vi "Projekt3.vi"() -> ()   [LabVIEW 2026]
uses:
  <vilib>/Utility/file.llb/Read Delimited Spreadsheet (string).vi
  <vilib>/Analysis/NI_AALBase.lvlib
panel:
  out "Approach3":dbl[](array[numeric])
  out "Approach2 Min":dbl[](array[numeric])
  out "Approach1 Max":dbl[](array[numeric])
  out "array w/ subset deleted":path[](array[path])
  out "All Files in Dir":path[](array[path])
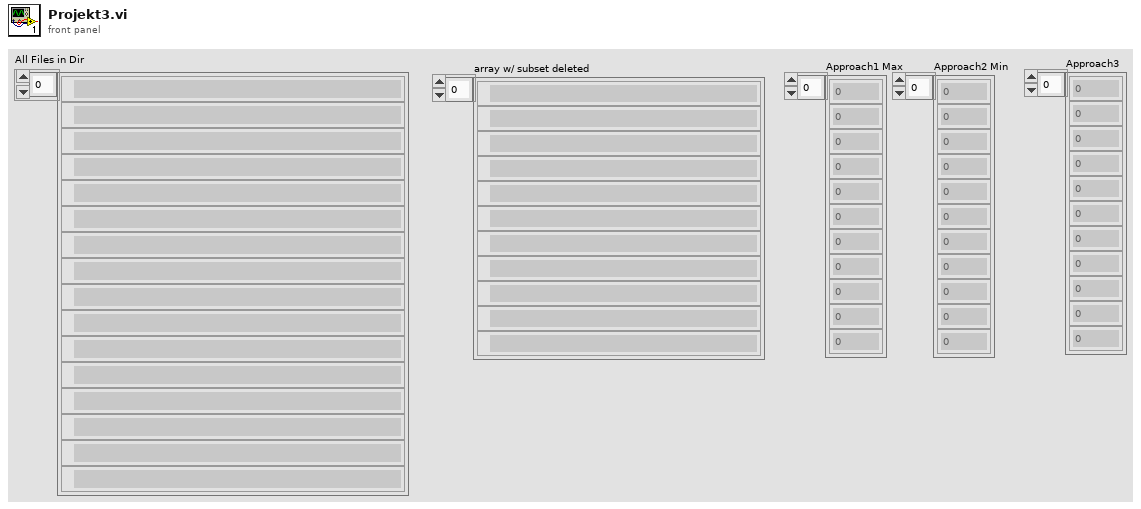
[diagram p1: front panel]
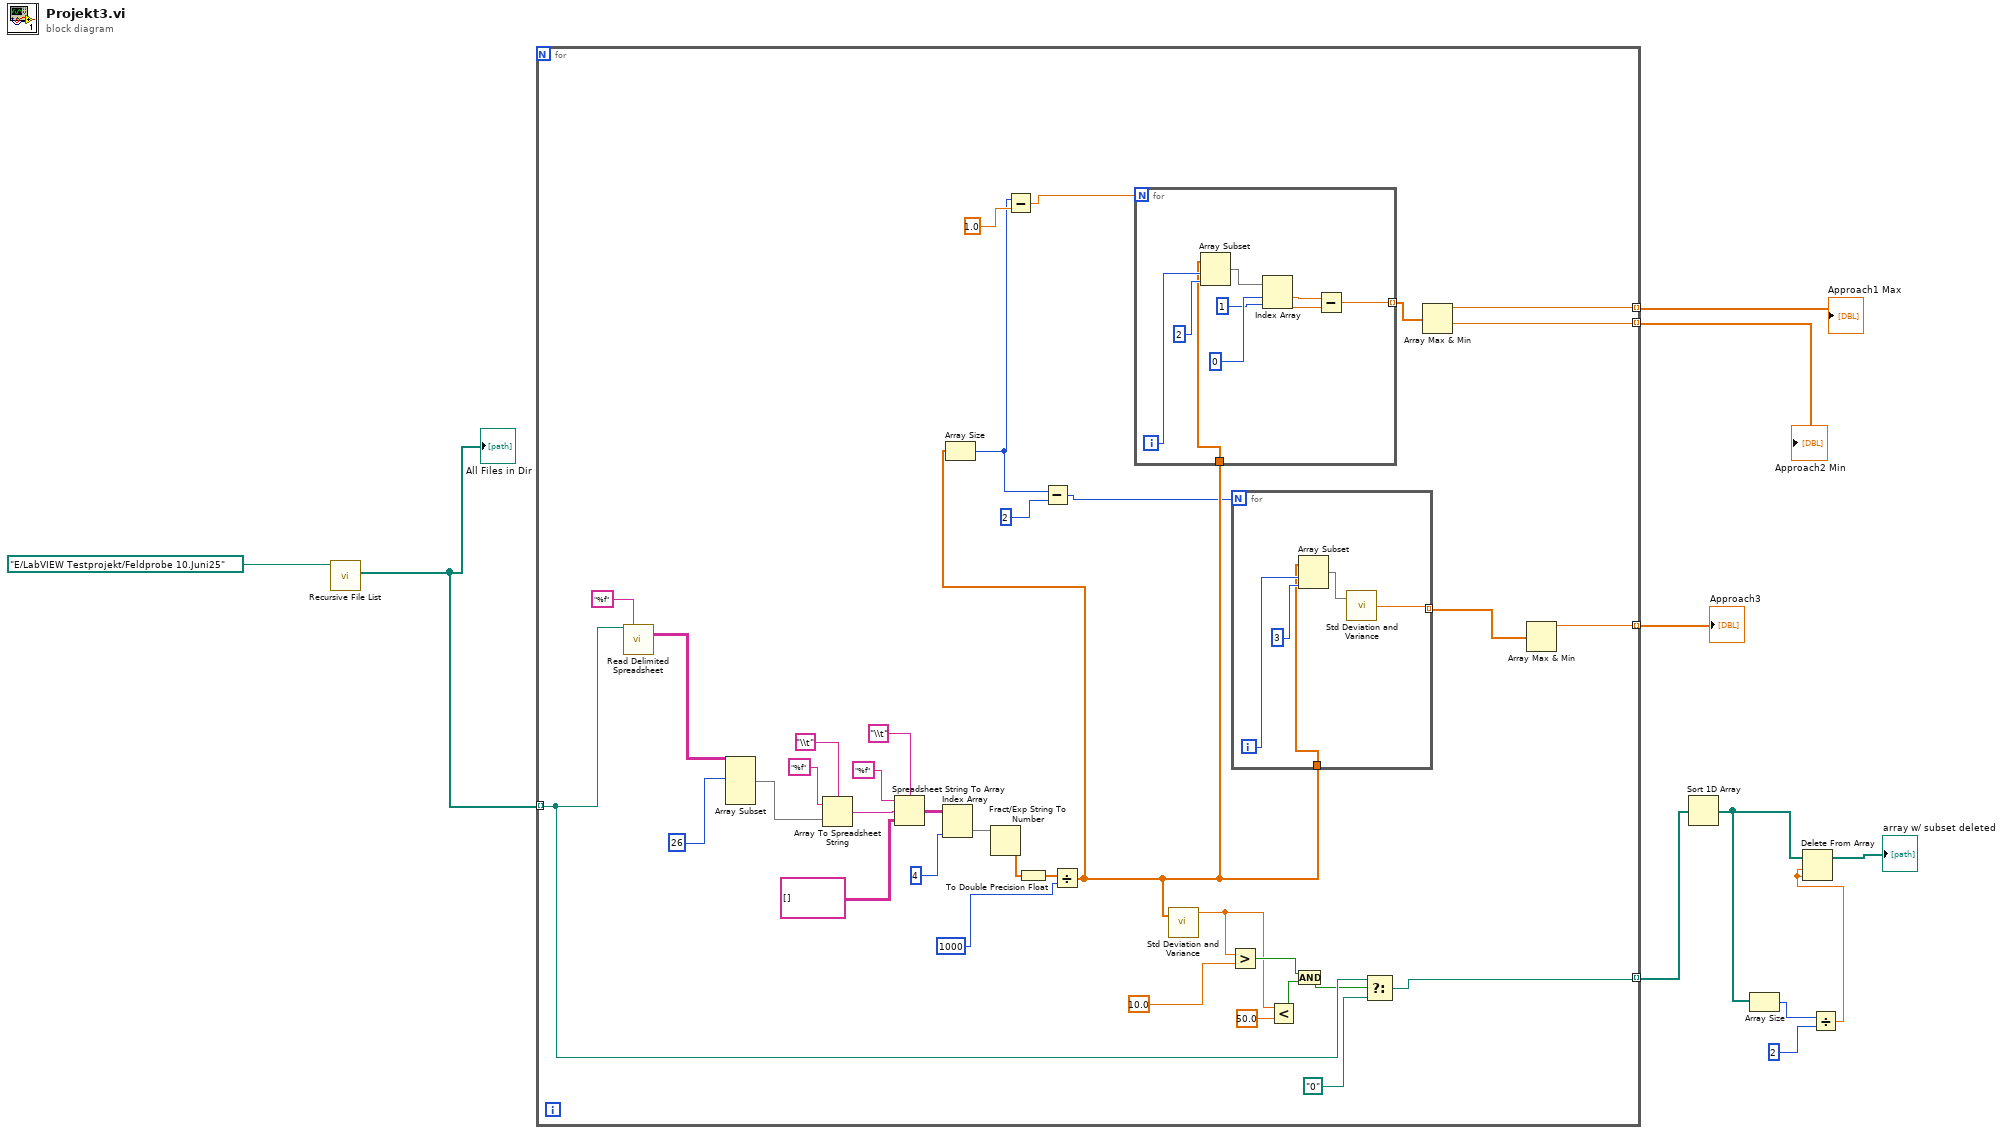
[diagram p0: block diagram]
diagram:
  n1 = call <vilib>:"Recursive File List.vi"("Folder Path"=path "E:/LabVIEW Testprojekt/Feldprobe 10.Juni25") -> ("All Files in Dir"=w10:path[])  [unwired: 6 in, 4 out]
  "All Files in Dir" <- w10
  n2 = for {
    tunnel: w10 -> [w31] mode=indexing
    tunnel: [w23] -> w9 mode=indexing
    tunnel: [w19] -> w3 mode=indexing
    tunnel: [w18] -> w2 mode=indexing
    tunnel: [w12] -> w1 mode=indexing
    n3 = call-poly <vilib>:"Read Delimited Spreadsheet.vi"("file path (dialog if empty)"=w31, "format (%s)"="%f") -> ("all rows"=w32:string[][])  [unwired: 8 in, 5 out]
    n4 = Array Subset(array=w32, index (row)=26 ("index")) -> (w44:string[][])  [unwired: 3 in]
    n5 = Array To Spreadsheet String(delimiter (Tab)="\\t", array=w44, 3:"%f" ("format string")) -> (spreadsheet string=w43:string)
    n6 = Spreadsheet String To Array(delimiter (Tab)="\\t", format string="%f", spreadsheet string=w43, array type (2D Dbl)=string[][] []) -> (array=w41:string[][])
    n7 = Index Array(array=w41, index (col)=4 ("disabled index (col)")) -> (element=w42:string[])  [unwired: 1 in]
    n8 = Fract/Exp String To Number(string=w42) -> (number=w46:dbl[])  [unwired: 3 in, 1 out]
    n9 = To Double Precision Float(number=w46) -> (double precision float=w45:dbl[])
    n10 = Divide(x=w45, y=1000) -> (x/y=w17:dbl[])
    n11 = Array Size(array=w17) -> (size(s)=w16:i32)
    n12 = Subtract(x=w16, y=1.0) -> (x-y=w21:dbl)
    n13 = Subtract(x=w16, y=2) -> (x-y=w14:i32)
    n14 = for {
      N: w21 -> [_]
      tunnel: w17 -> [w53]
      tunnel: [w55] -> w20 mode=indexing
      i -> [w54]
      n15 = Array Subset(array=w53, index=w54, length=2) -> (w60:dbl[])
      n16 = Index Array(array=w60, index #1=0 ("index"), index #2=1 ("index")) -> (element #1=w57:dbl, element #2=w56:dbl)
      n17 = Subtract(x=w57, y=w56) -> (x-y=w55:dbl)
    }
    n18 = call <vilib>:"Std Deviation and Variance.vi"("X"=w17) -> ("mean"=w27:dbl)  [unwired: 1 in, 2 out]
    n19 = Greater?(x=w27, y=10.0) -> (0:w29:bool)
    n20 = for {
      N: w14 -> [_]
      tunnel: w17 -> [w50]
      tunnel: [w48] -> w13 mode=indexing
      i -> [w51]
      n21 = Array Subset(array=w50, index=w51, length=3) -> (w49:dbl[])
      n22 = call <vilib>:"Std Deviation and Variance.vi"("X"=w49) -> ("standard deviation"=w48:dbl)  [unwired: 1 in, 2 out]
    }
    n23 = Less?(x=w27, y=50.0) -> (x < y?=w28:bool)
    n24 = And(x=w29, y=w28) -> (x .and. y?=w25:bool)
    n25 = Select(t=w31, s=w25, f=path "0") -> (s? t:f=w23:path)
    n26 = Array Max & Min(array=w20) -> (max value=w19:dbl, min value=w18:dbl)  [unwired: 2 out]
    n27 = Array Max & Min(array=w13) -> (max value=w12:dbl)  [unwired: 3 out]
  }
  "Approach1 Max" <- w3
  "Approach2 Min" <- w2
  "Approach3" <- w1
  n28 = Sort 1D Array(array=w9) -> (sorted array=w8:path[])
  n29 = Array Size(array=w8) -> (size(s)=w7:i32)
  n30 = Divide(x=w7, y=2) -> (x/y=w5:dbl)
  n31 = Delete From Array(array=w8, length=w5, index=w5) -> (array with subset deleted=→"array w/ subset deleted":path[])  [unwired: 1 out]
